vi "SetupCallBackEvents.vi"(8 "error in (no error)":errorcluster, 11 "DataGridView in":refnum<class "DataGridView.lvclass">) -> (0 "error out":errorcluster, 3 "DataGridView out":refnum<class "DataGridView.lvclass">)   [LabVIEW 2020, in "DataGrid.lvlib" / "DataGridView.lvclass"]
doc: "Callbacks are used to tie the .net grid events to the labview event structure and this VI sets the callback VIs up for each of the possible events for the grid class."
uses:
  DataGridView.lvclass
  Events/Abstract EVENT/Abstract EVENT.lvclass
  DataGridView.lvclass/DataGridView.ctl
  Properties/Read DataGridView.vi
  System.Windows.Forms
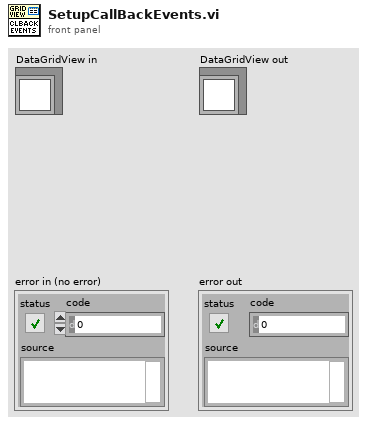
[diagram p1: front panel]
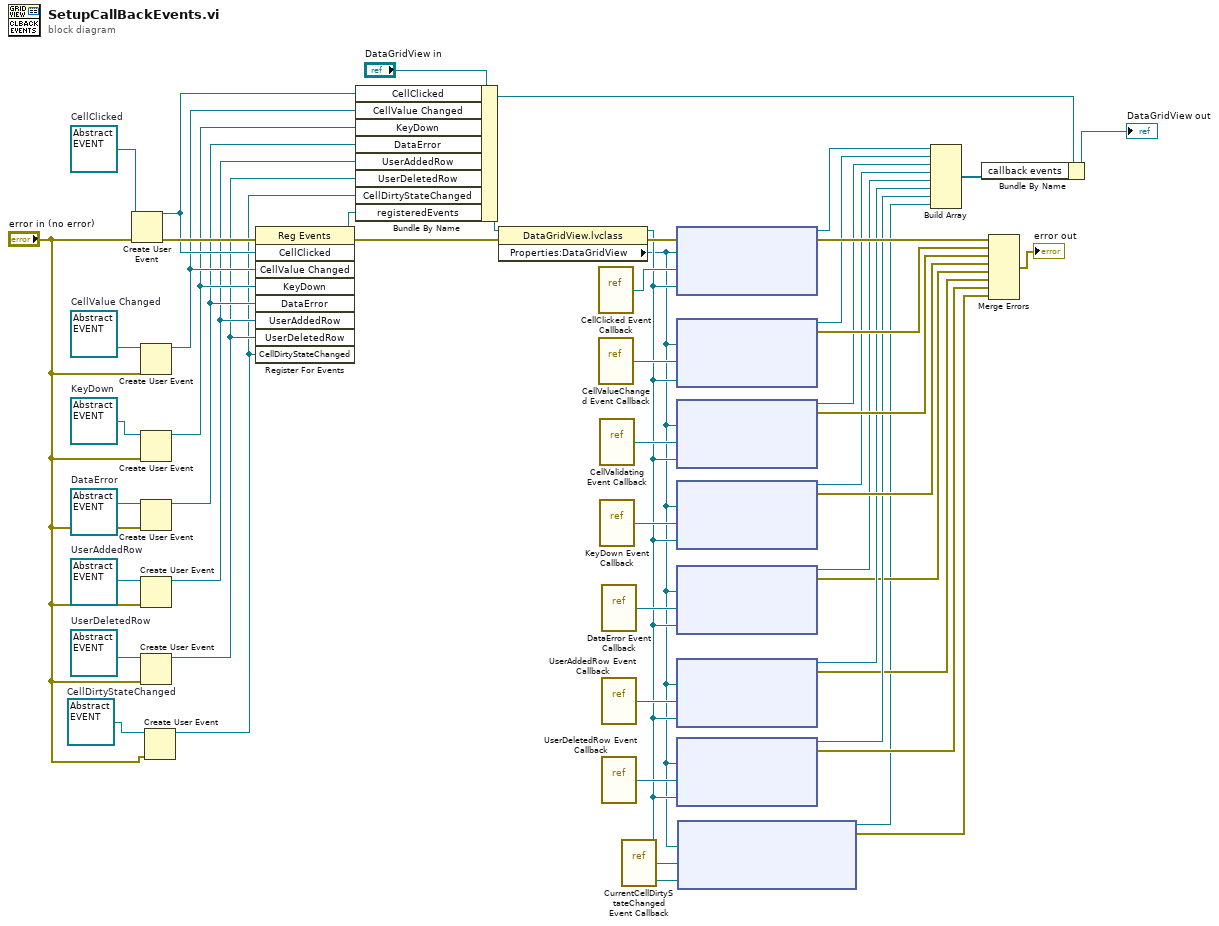
[diagram p0: block diagram]
diagram:
  w2 = refnum<class "Abstract EVENT.lvclass"> refnum  # CellDirtyStateChanged
  w26 = refnum<class "Abstract EVENT.lvclass"> refnum  # UserDeletedRow
  w28 = refnum<class "Abstract EVENT.lvclass"> refnum  # UserAddedRow
  w27 = refnum<class "Abstract EVENT.lvclass"> refnum  # DataError
  w33 = refnum<class "Abstract EVENT.lvclass"> refnum  # KeyDown
  w37 = refnum<class "Abstract EVENT.lvclass"> refnum  # CellClicked
  w38 = refnum<class "Abstract EVENT.lvclass"> refnum  # CellValue Changed
  n1 = Create User Event(user event datatype=w37, error in="error in (no error)") -> (user event=w17:refnum<user-event>, error out=w50:errorcluster)
  n2 = Create User Event(user event datatype=w38, error in="error in (no error)") -> (user event=w16:refnum<user-event>)  [unwired: 1 out]
  n3 = Create User Event(user event datatype=w33, error in="error in (no error)") -> (user event=w15:refnum<user-event>)  [unwired: 1 out]
  n4 = Create User Event(user event datatype=w27, error in="error in (no error)") -> (user event=w14:refnum<user-event>)  [unwired: 1 out]
  n5 = Create User Event(user event datatype=w28, error in="error in (no error)") -> (user event=w13:refnum<user-event>)  [unwired: 1 out]
  n6 = Create User Event(user event datatype=w26, error in="error in (no error)") -> (user event=w12:refnum<user-event>)  [unwired: 1 out]
  n7 = Create User Event(user event datatype=w2, error in="error in (no error)") -> (user event=w8:refnum<user-event>)  [unwired: 1 out]
  n8 = register-events(error in=w50, w17, w16, w15, w14, w13, w12, w8) -> (reference out=w7:refnum<event-registration>, error out=w48:errorcluster)  [unwired: 1 in]
  n9 = Bundle By Name(cluster="DataGridView in", "CellClicked"=w17, "CellValue Changed"=w16, "KeyDown"=w15, "DataError"=w14, "UserAddedRow"=w13, "UserDeletedRow"=w12, "CellDirtyStateChanged"=w8, "registeredEvents"=w7) -> (w10:refnum<class "DataGridView.lvclass">)
  n10 = property class="DataGridView.lvclass"(reference=w10, error in=w48) -> (reference out=w6:refnum<class "DataGridView.lvclass">, error out=w49:errorcluster, "Properties:DataGridView"=w5:refnum<k24>)
  n11 = vi-ref "CellClicked Event Callback.vi"() -> ("vi reference"=w47:refnum<vi>)
  n12 = vi-ref "CellValueChanged Event Callback.vi"() -> ("vi reference"=w19:refnum<vi>)
  n13 = vi-ref "CellValidating Event Callback.vi"() -> ("vi reference"=w18:refnum<vi>)
  n14 = vi-ref "KeyDown Event Callback.vi"() -> ("vi reference"=w32:refnum<vi>)
  n15 = vi-ref "DataError Event Callback.vi"() -> ("vi reference"=w31:refnum<vi>)
  n16 = vi-ref "UserAddedRow Event Callback.vi"() -> ("vi reference"=w30:refnum<vi>)
  n17 = vi-ref "UserDeletedRow Event Callback.vi"() -> ("vi reference"=w29:refnum<vi>)
  n18 = vi-ref "CurrentCellDirtyStateChanged Event Callback.vi"() -> ("vi reference"=w1:refnum<vi>)
  n19 = node(w49, w5, w47, w6) -> (w42:refnum<k27>, w46:errorcluster)  [unwired: 1 in]
  n20 = node(w5, w19, w6) -> (w43:refnum<k27>, w45:errorcluster)  [unwired: 2 in]
  n21 = node(w5, w18, w6) -> (w41:refnum<k27>, w36:errorcluster)  [unwired: 2 in]
  n22 = node(w5, w32, w6) -> (w34:refnum<k27>, w35:errorcluster)  [unwired: 2 in]
  n23 = node(w5, w31, w6) -> (w25:refnum<k27>, w22:errorcluster)  [unwired: 2 in]
  n24 = node(w5, w30, w6) -> (w24:refnum<k27>, w21:errorcluster)  [unwired: 2 in]
  n25 = node(w5, w29, w6) -> (w23:refnum<k27>, w20:errorcluster)  [unwired: 2 in]
  n26 = node(w5, w1, w6) -> (w4:refnum<k27>, w3:errorcluster)  [unwired: 2 in]
  n27 = Build Array(w42, w43, w41, w34, w25, w24, w23, w4) -> (w39:refnum<k27>[])
  n28 = Bundle By Name(cluster=w10, "callback events"=w39) -> (→"DataGridView out":refnum<class "DataGridView.lvclass">)
  n29 = Merge Errors(w46, w45, w36, w35, w22, w21, w20, w3) -> (→"error out":errorcluster)
